vi "9215 4Ch Analog Input.vi"(1 "9215 I/O":T1={"9215 AI0"="NI 9215/AI0", "9215 AI1"="NI 9215/AI1", "9215 AI2"="NI 9215/AI2", "9215 AI3"="NI 9215/AI3"}) -> (0 "Packets":u64[](array[numeric]))   [LabVIEW 2010]
uses:
  <vilib>/eio/EIONode/EIONode.xnode
  <vilib>/rvi/eio/nirviEIOImplementation/nirviEIOImplementation.xnode
  <vilib>/rvi/eio/common/nirviEmuClasses.ctl
  <vilib>/rvi/eio/common/nirviEmuTemplateMethod_noerrors.vi
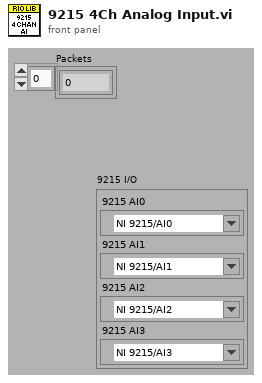
[diagram p1: front panel]
types:
  T1 = cluster{"9215 AI0":refnum<k21>, "9215 AI1":refnum<k21>, "9215 AI2":refnum<k21>, "9215 AI3":refnum<k21>}
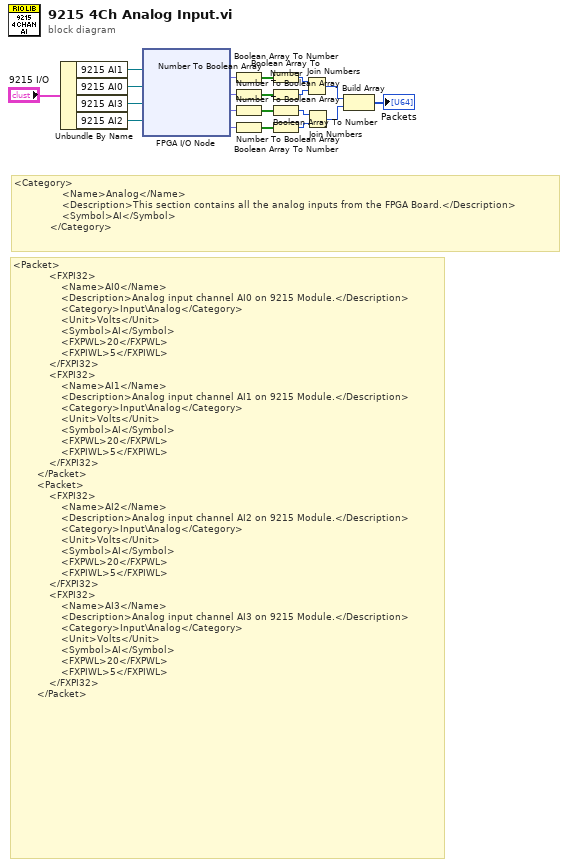
[diagram p0: block diagram]
diagram:
  # "<Category>\n                <Name>Analog</Name>\n                <Description>This section contains all the analog inputs from the FPGA Board.</Description>\n                <Symbol>AI</Symbol>\n            </Category>"
  # "<Packet>\n            <FXPI32>\n                <Name>AI0</Name>\n                <Description>Analog input channel AI0 on 9215 Module.</Description>\n                <Category>Input\\Analog</Category>\n                <Unit>Volts</Unit>\n                <Symbol>AI</Symbol>\n                <FXPWL>20</FXPWL>\n                <FXPIWL>5</FXPIWL>\n            </FXPI32>\n            <FXPI32>\n                <Name>AI1</Name>\n                <Description>Analog input channel AI1 on 9215 Module.</Description>\n                <Category>Input\\Analog</Category>\n                <Unit>Volts</Unit>\n                <Symbol>AI</Symbol>\n                <FXPWL>20</FXPWL>\n                <FXPIWL>5</FXPIWL>\n            </FXPI32>\n        </Packet>\n        <Packet>\n            <FXPI32>\n                <Name>AI2</Name>\n                <Description>Analog input channel AI2 on 9215 Module.</Description>\n                <Category>Input\\Analog</Category>\n                <Unit>Volts</Unit>\n                <Symbol>AI</Symbol>\n                <FXPWL>20</FXPWL>\n                <FXPIWL>5</FXPIWL>\n            </FXPI32>\n            <FXPI32>\n                <Name>AI3</Name>\n                <Description>Analog input channel AI3 on 9215 Module.</Description>\n                <Category>Input\\Analog</Category>\n                <Unit>Volts</Unit>\n                <Symbol>AI</Symbol>\n                <FXPWL>20</FXPWL>\n                <FXPIWL>5</FXPIWL>\n            </FXPI32>\n        </Packet>"
  n1 = Unbundle By Name("9215 I/O") -> ("9215 AI1"=w1:refnum<k21>, "9215 AI0"=w4:refnum<k21>, "9215 AI3"=w2:refnum<k21>, "9215 AI2"=w5:refnum<k21>)
  n2 = xnode "FPGA I/O Node"("FPGA I/O In"=w1, "FPGA I/O In"=w4, "FPGA I/O In"=w2, "FPGA I/O In"=w5) -> ("I/O Item"=w11:fxp<+/-,20,5>, "I/O Item"=w13:fxp<+/-,20,5>, "I/O Item"=w3:fxp<+/-,20,5>, "I/O Item"=w12:fxp<+/-,20,5>)  [unwired: 4 out]
  n3 = Number To Boolean Array(number=w11) -> (Boolean array=w7:bool[])
  n4 = Number To Boolean Array(number=w13) -> (Boolean array=w8:bool[])
  n5 = Number To Boolean Array(number=w3) -> (Boolean array=w10:bool[])
  n6 = Number To Boolean Array(number=w12) -> (Boolean array=w9:bool[])
  n7 = Boolean Array To Number(Boolean array=w7) -> (number=w14:u32)
  n8 = Boolean Array To Number(Boolean array=w8) -> (number=w15:u32)
  n9 = Boolean Array To Number(Boolean array=w10) -> (number=w16:u32)
  n10 = Boolean Array To Number(Boolean array=w9) -> (number=w17:u32)
  n11 = Join Numbers(hi=w14, lo=w15) -> ((hi.lo)=w18:u64)
  n12 = Join Numbers(hi=w16, lo=w17) -> ((hi.lo)=w19:u64)
  n13 = Build Array(w18, w19) -> (→"Packets":u64[])
